vi "A軸回home_function2.vi"(7 "A¶b Home_action":T1, 8 "error in (no error)":errorcluster) -> (0 "error out":errorcluster)   [LabVIEW 2014]
uses:
  axis motion function.ctl
  global/Global.vi
panel:
  out "state":u8
  # "A軸是彈簧的夾爪"
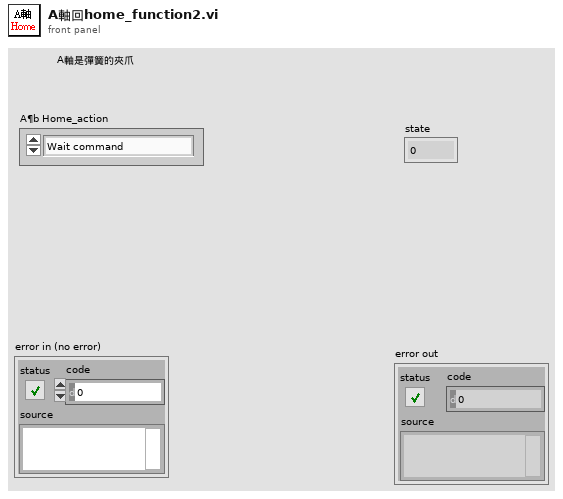
[diagram p1: front panel]
types:
  T1 = typedef "A¶b home_action.ctl" = enum16{"Wait command", "Config phi motor", "Start phi homing", "確認 phi homing done", "error"}
  T2 = typedef "axis motion function.ctl" = enum16{"Wait command", "Axis_S motion", "Axis_P motion", "Axis_Motion_Satus_CK", "Axis _S position CK", "Axis_P position CK", "finish", "error"}
  T3 = typedef "home function.ctl" = enum16{"Wait command", "Config X home mode_7", "Start X homing_7", "確認 X homing_7 done", "Config Y home mode_7", "Start Y homing_7", "確認 Y homing_7 done", "Config Z home mode_7", "Start Z homing_7", "確認 Z homing_7 done", "Config phi motor", "Start phi homing", "確認 phi homing done", "finish", "error"}
  T4 = typedef "軸參數記錄.ctl" = cluster{"X軸取料位":dbl, "X¶bCCD¦ì":dbl, "X軸影像異常排料位":dbl, "X軸迴轉缸位":dbl, "裝完料區已可安全取料位":dbl, "A軸取料角":dbl, "A¶bCCD¨¤":dbl, "B軸取料角":dbl, "B¶bCCD¨¤":dbl, "軸控參數PATH":path, "CCD左連續失敗報警次數":u8, "CCD右連續失敗報警次數":u8, "連續組裝失敗報警次數":u8, "ABVL/VH":i32, "XVL/VH":i32, "AB加速度":i32, "X加速度":i32, "home-XVL/VH":i32, "home-ABVL/VH":i32}
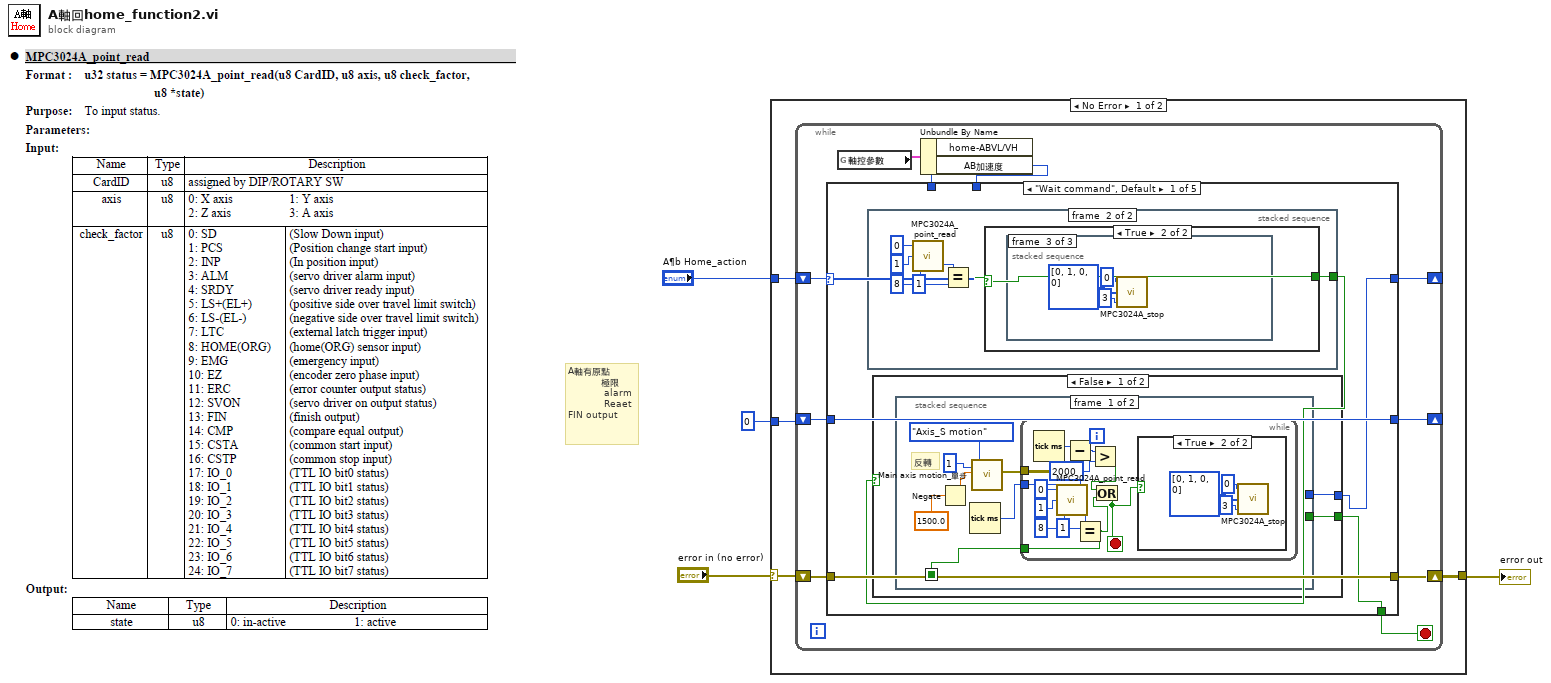
[diagram p0: block diagram]
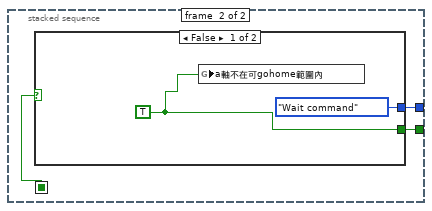
[diagram p3: hidden frame]
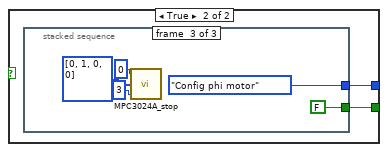
[diagram p4: hidden frame]
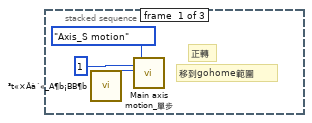
[diagram p5: hidden frame]
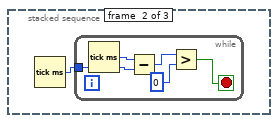
[diagram p6: hidden frame]
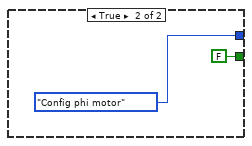
[diagram p7: hidden frame]
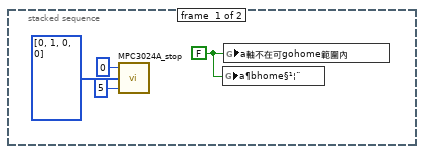
[diagram p8: hidden frame]
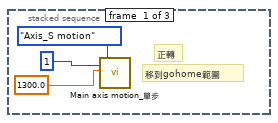
[diagram p10: hidden frame]
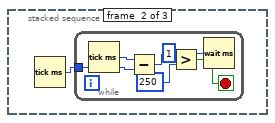
[diagram p11: hidden frame]
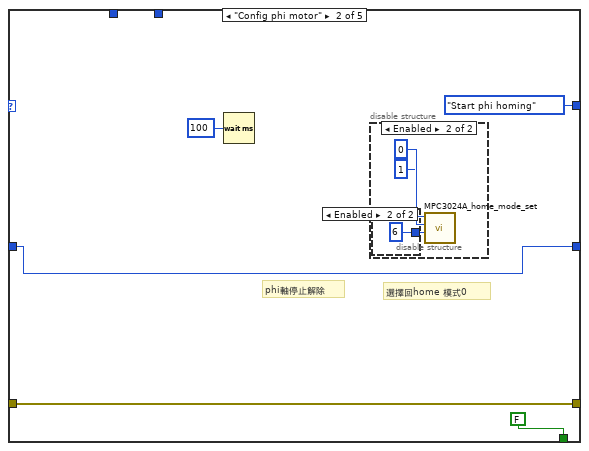
[diagram p12: hidden frame]
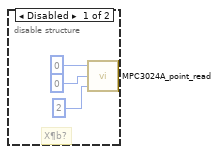
[diagram p13: hidden frame]
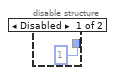
[diagram p14: hidden frame]
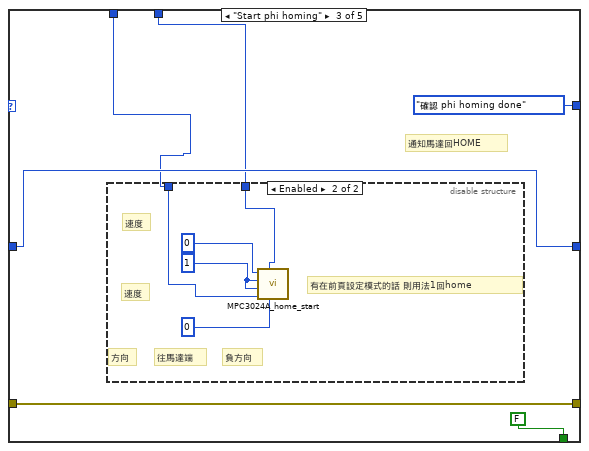
[diagram p15: hidden frame]
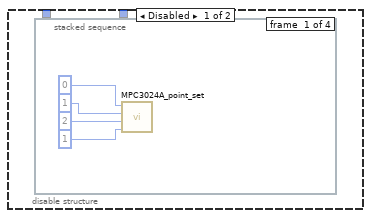
[diagram p16: hidden frame]
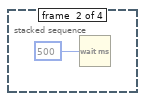
[diagram p17: hidden frame]
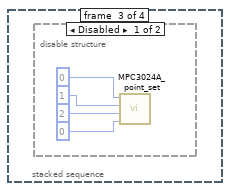
[diagram p18: hidden frame]
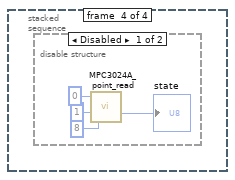
[diagram p20: hidden frame]
diagram:
  # "A軸有原點\n           極限\n            alarm\n            Reaet\nFIN output"
  n1 = case shown="No Error" "error in (no error)" {
    selector: "error in (no error)" -> [w7 w187]
    tunnel: [w6 w187] -> w3
    tunnel: "A¶b Home_action" -> [w8 _]
    tunnel: 0 -> [w5 _]
    frame No Error {
      n2 = while {
        shift-right: [w17] -> _
        shift-left: w8 -> [w18]
        shift-right: [w14] -> w6
        shift-left: w7 -> [w15]
        shift-right: [w12] -> _
        shift-left: w5 -> [w13]
        stop <- w16 stop-if-true
        n3 = global read "Global.vi" "軸控參數"() -> (w11:T4)
        n4 = Unbundle By Name(w11) -> ("home-ABVL/VH"=w10:i32, "AB加速度"=w9:i32)
        n5 = case shown="\"Wait command\", Default" w18 {
          tunnel: [w20 A¶b_home_action."Start phi homing" ("A¶b Home_action") A¶b_home_action."確認 phi homing done" ("A¶b Home_action") w134 _] -> w17
          tunnel: [w19 FALSE FALSE w135 TRUE] -> w16
          tunnel: w15 -> [w23 w98 w114 _ w179]
          tunnel: [w23 w98 w114 w136 w179] -> w14
          tunnel: w13 -> [w22 w97 w112 w138 w180]
          tunnel: [w22 w97 w112 w137 w180] -> w12
          tunnel: w10 -> [_ _ w111 _ _]
          tunnel: w9 -> [_ _ w110 _ _]
          frame "Wait command", Default {
            n6 = stacked-sequence {
              tunnel: [_ w75] -> w21
              frame #0 {
                w71 = FALSE ("a軸不在可gohome範圍內")
                n7 = call "MPC3024A_stop.vi"("Tdec_ms"=u32 5, "axis[4]"=u8[] [0, 1, 0, 0], "CardID"=u8 0) -> ()  [unwired: 1 out]
                n8 = global write "Global.vi" "a¶bhome§¹¦¨"(w71) -> ()
                n9 = global write "Global.vi" "a軸不在可gohome範圍內"(w71) -> ()
              }
              frame #1 {
                n10 = call "MPC3024A_point_read.vi"("check_factor"=u8 8, "axis"=u8 1, "CardID"=u8 0) -> ("state"=w78:u8)  [unwired: 1 out]
                n11 = Equal?(x=w78, y=u8 1) -> (x = y?=w76:bool)
                n12 = case shown="True" w76 {
                  selector: w76 -> [w82 w83]
                  tunnel: [w82 w83] -> w75
                  frame False {
                  }
                  frame True {
                    n13 = stacked-sequence {
                      frame #0 {
                        # "移到gohome範圍"
                        # "正轉"
                        n14 = call "Main axis motion_單步.vi"("axis"=u8 1, "VL/VH"=1300.0 ("轉速(rpm)"), "Axis motion function"=axis_motion_function."Axis_S motion") -> ()  [unwired: 14 in, 3 out]
                      }
                      frame #1 {
                        n15 = Tick Count (ms)() -> (millisecond timer value=w87:u32)
                        n16 = while {
                          tunnel: w87 -> [w92]
                          stop <- w89 stop-if-true
                          n17 = Tick Count (ms)() -> (millisecond timer value=w93:u32)
                          n18 = Subtract(x=w93, y=w92) -> (x-y=w91:u32)
                          n19 = Greater?(x=w91, y=u32 250) -> (0:w89:bool)
                          n20 = Wait (ms)(milliseconds to wait=u32 1) -> ()  [unwired: 1 out]
                        }
                      }
                      frame #2 {
                        n21 = call "MPC3024A_stop.vi"("Tdec_ms"=u32 3, "axis[4]"=u8[] [0, 1, 0, 0], "CardID"=u8 0) -> ()  [unwired: 1 out]
                      }
                    }
                  }
                }
              }
            }
            n22 = case shown="False" w21 {
              tunnel: [w25 A¶b_home_action."Config phi motor" ("A¶b Home_action")] -> w20
              tunnel: [w24 FALSE] -> w19
              frame False {
                n23 = stacked-sequence {
                  seq-local: [w27 _] -> [_ w50]
                  tunnel: [_ w49] -> w25
                  tunnel: [_ w48] -> w24
                  frame #0 {
                    # "反轉"
                    n24 = Negate(x=1500.0 ("轉速(rpm)")) -> (-x=w32:dbl)
                    n25 = Tick Count (ms)() -> (millisecond timer value=w29:u32)
                    n26 = call "Main axis motion_單步.vi"("axis"=u8 1, "VL/VH"=w32, "Axis motion function"=axis_motion_function."Axis_S motion") -> ("error out"=w28:errorcluster)  [unwired: 14 in, 2 out]
                    n27 = while {
                      tunnel: w29 -> [w43]
                      tunnel: w28 -> [_]
                      tunnel: [w33] -> w27
                      stop <- w34 stop-if-true
                      n28 = Tick Count (ms)() -> (millisecond timer value=w44:u32)
                      n29 = call "MPC3024A_point_read.vi"("check_factor"=u8 8, "axis"=u8 1, "CardID"=u8 0) -> ("state"=w39:u8)  [unwired: 1 out]
                      n30 = Subtract(x=w44, y=w43) -> (x-y=w42:u32)
                      n31 = Equal?(x=w39, y=u8 1) -> (x = y?=w33:bool)
                      n32 = Greater?(x=w42, y=u32 2000) -> (0:w35:bool)
                      n33 = Or(x=w35, y=w33) -> (x .or. y?=w34:bool)
                      n34 = case shown="True" w34 {
                        frame False {
                        }
                        frame True {
                          n35 = call "MPC3024A_stop.vi"("Tdec_ms"=u32 3, "axis[4]"=u8[] [0, 1, 0, 0], "CardID"=u8 0) -> ()  [unwired: 1 out]
                        }
                      }
                    }
                  }
                  frame #1 {
                    n36 = case shown="False" w50 {
                      tunnel: [A¶b_home_action."Wait command" ("A¶b Home_action") w54] -> w49
                      tunnel: [w51 w53] -> w48
                      frame False {
                        w51 = TRUE
                        n37 = global write "Global.vi" "a軸不在可gohome範圍內"(w51) -> ()
                      }
                      frame True {
                        n38 = stacked-sequence {
                          tunnel: [_ _ A¶b_home_action."Config phi motor" ("A¶b Home_action")] -> w54
                          tunnel: [_ _ FALSE] -> w53
                          frame #0 {
                            # "移到gohome範圍"
                            # "正轉"
                            n39 = call "³t«×Âà´«_A¶b¡BB¶b.vi"() -> ("轉速(pps)"=w57:i32)  [unwired: 11 in]
                            n40 = call "Main axis motion_單步.vi"("axis"=u8 1, "VL/VH"=w57, "Axis motion function"=axis_motion_function."Axis_S motion") -> ()  [unwired: 14 in, 3 out]
                          }
                          frame #1 {
                            n41 = Tick Count (ms)() -> (millisecond timer value=w58:u32)
                            n42 = while {
                              tunnel: w58 -> [w62]
                              stop <- w59 stop-if-true
                              n43 = Tick Count (ms)() -> (millisecond timer value=w63:u32)
                              n44 = Subtract(x=w63, y=w62) -> (x-y=w61:u32)
                              n45 = Greater?(x=w61, y=u32 0) -> (0:w59:bool)
                            }
                          }
                          frame #2 {
                            n46 = call "MPC3024A_stop.vi"("Tdec_ms"=u32 3, "axis[4]"=u8[] [0, 1, 0, 0], "CardID"=u8 0) -> ()  [unwired: 1 out]
                          }
                        }
                      }
                    }
                  }
                }
              }
              frame True {
              }
            }
          }
          frame "Config phi motor" {
            # "選擇回home 模式0"
            # "phi軸停止解除"
            n47 = Wait (ms)(milliseconds to wait=u32 100) -> ()  [unwired: 1 out]
            n48 = disable-structure shown="Enabled" {
              frame Disabled {
                # "X¶b?"
                n49 = call "MPC3024A_point_read.vi"("check_factor"=u8 2, "axis"=u8 0, "CardID"=u8 0) -> ()  [unwired: 2 out]
              }
              frame Enabled {
                n50 = disable-structure shown="Enabled" {
                  disable-tunnel: [u8 1 ("mode") u8 6 ("mode")] -> w105
                  frame Disabled {
                  }
                  frame Enabled {
                  }
                }
                n51 = call "MPC3024A_home_mode_set.vi"("mode"=w105, "axis"=u8 1, "CardID"=u8 0) -> ()  [unwired: 1 in, 1 out]
              }
            }
          }
          frame "Start phi homing" {
            # "通知馬達回HOME"
            n52 = disable-structure shown="Enabled" {
              disable-tunnel: w111 -> [_ w131]
              disable-tunnel: w110 -> [_ w129]
              frame Disabled {
                n53 = stacked-sequence {
                  frame #0 {
                    n54 = call "MPC3024A_point_set.vi"("on_off"=u8 1, "check_factor"=u8 2, "axis"=u8 1, "CardID"=u8 0) -> ()  [unwired: 1 out]
                  }
                  frame #1 {
                    n55 = Wait (ms)(milliseconds to wait=u32 500) -> ()  [unwired: 1 out]
                  }
                  frame #2 {
                    n56 = disable-structure shown="Disabled" {
                      frame Disabled {
                        n57 = call "MPC3024A_point_set.vi"("on_off"=u8 0, "check_factor"=u8 2, "axis"=u8 1, "CardID"=u8 0) -> ()  [unwired: 1 out]
                      }
                      frame Enabled {
                      }
                    }
                  }
                  frame #3 {
                    n58 = disable-structure shown="Disabled" {
                      frame Disabled {
                        n59 = call "MPC3024A_point_read.vi"("check_factor"=u8 8, "axis"=u8 1, "CardID"=u8 0) -> ("state"=→"state":u8)  [unwired: 1 out]
                      }
                      frame Enabled {
                      }
                    }
                  }
                }
              }
              frame Enabled {
                w130 = u8 1 ("axis")
                # "負方向"
                # "往馬達端"
                # "有在前頁設定模式的話 則用法1回home"
                # "速度"
                # "速度"
                # "方向"
                n60 = call "MPC3024A_home_start.vi"("direction"=u8 0, "Tacc_ms"=w129, "VH"=w131, "VL"=w130, "axis"=w130, "CardID"=u8 0) -> ()  [unwired: 1 out]
              }
            }
          }
          frame "確認 phi homing done" {
            n61 = disable-structure shown="Enabled" {
              disable-tunnel: [w142 w147] -> w140
              frame Disabled {
                n62 = call "MPC3024A_point_read.vi"("check_factor"=u8 8, "axis"=u8 1, "CardID"=u8 0) -> ("state"=w146:u8)  [unwired: 1 out]
                n63 = Equal?(x=w146, y=u8 1) -> (x = y?=w142:bool)
              }
              frame Enabled {
                n64 = call "MPC3024A_motion_status_read.vi"("check_factor"=u8 0, "axis"=u8 1, "CardID"=u8 0) -> ("ret_fig"=w148:u8)  [unwired: 1 out]
                n65 = Equal?(x=w148, y=u8 1) -> (x = y?=w147:bool)
              }
            }
            n66 = Wait (ms)(milliseconds to wait=u32 100) -> ()  [unwired: 1 out]
            n67 = case shown="False" w140 {
              selector: w140 -> [_ w168]
              tunnel: w138 -> [w161 _]
              tunnel: [w159 0] -> w137
              tunnel: [w157 errorcluster {"status"=FALSE, "code"=0, "source"=""} ("error in (no error)")] -> w136
              tunnel: [w154 w168] -> w135
              tunnel: [w153 _] -> w134
              frame False {
                n68 = Increment(x=w161) -> (x+1=w158:i32)
                n69 = Wait (ms)(milliseconds to wait=u32 100) -> ()  [unwired: 1 out]
                n70 = Less?(x=w158, y=100) -> (x < y?=w155:bool)
                n71 = Not(x=w155) -> (.not. x?=w154:bool)
                n72 = case shown="True" w155 {
                  tunnel: [0 w167] -> w159
                  tunnel: w158 -> [_ w167]
                  tunnel: [errorcluster {"status"=TRUE, "code"=0, "source"="A軸回home失敗"} ("error in (no error)") errorcluster {"status"=FALSE, "code"=0, "source"=""} ("error in (no error)")] -> w157
                  tunnel: [A¶b_home_action."error" ("A¶b Home_action") A¶b_home_action."確認 phi homing done" ("A¶b Home_action")] -> w153
                  frame False {
                  }
                  frame True {
                  }
                }
              }
              frame True {
                n73 = disable-structure shown="Enabled" {
                  frame Enabled {
                    n74 = call "MPC3024A_current_position_set.vi"("current_posi"=0, "axis"=u8 1, "CardID"=u8 0) -> ()  [unwired: 1 out]
                  }
                  frame Disabled {
                  }
                }
                n75 = disable-structure shown="Disabled" {
                  frame Disabled {
                    n76 = call "MPC3024A_FB_counter_set.vi"("value"=0, "axis"=u8 3, "CardID"=u8 0) -> ()  [unwired: 1 out]
                  }
                  frame Enabled {
                  }
                }
                n77 = disable-structure shown="Disabled" {
                  disable-tunnel: [home_function."finish" ("Home function") _] -> _
                  frame Disabled {
                  }
                  frame Enabled {
                  }
                }
              }
            }
          }
          frame "error" {
            n78 = disable-structure shown="Enabled" {
              frame Disabled {
                # "各軸STOP"
                n79 = call "MPC3024A_stop.vi"("Tdec_ms"=u32 10, "axis[4]"=u8[] [1, 1, 1, 1], "CardID"=u8 0) -> ()  [unwired: 1 out]
              }
              frame Enabled {
                n80 = call "MPC3024A_stop.vi"("Tdec_ms"=u32 10, "axis[4]"=u8[] [0, 1, 0, 0], "CardID"=u8 0) -> ()  [unwired: 1 out]
              }
            }
          }
        }
      }
    }
    frame Error {
    }
  }
  "error out" <- w3
